vi "BinaryFile_input_output.vi"() -> ()   [LabVIEW 2018]
panel:
  out "웨이브폼 그래프":dbl[](graph)
  out "웨이브폼 차트":dbl(graph)
  in  "정지 버튼 2":bool
  in  "파일 경로(대화 상자 사용)":path
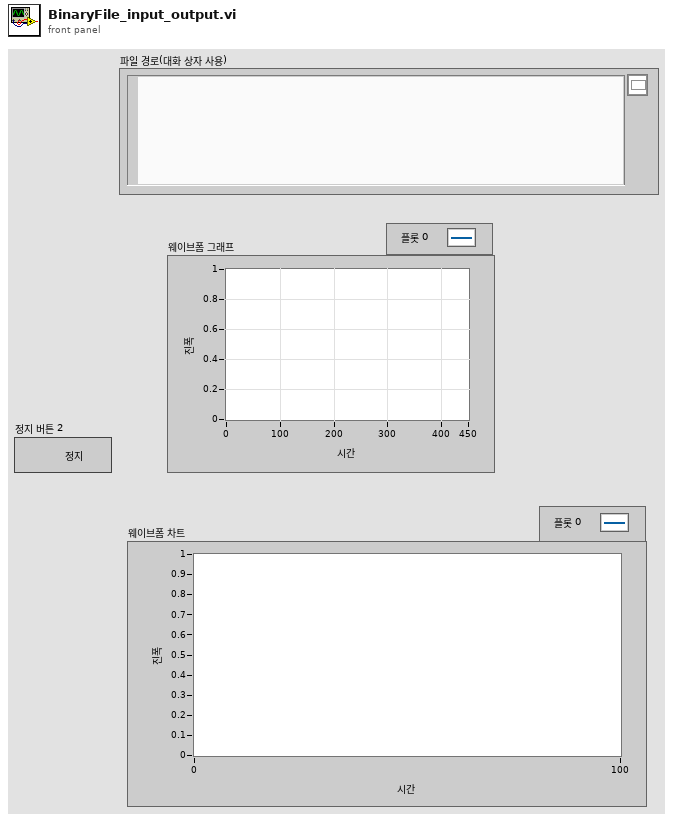
[diagram p1: front panel]
types:
  T1 = enum16{"open", "replace", "create", "open or create", "replace or create", "replace or create with confirmation"}
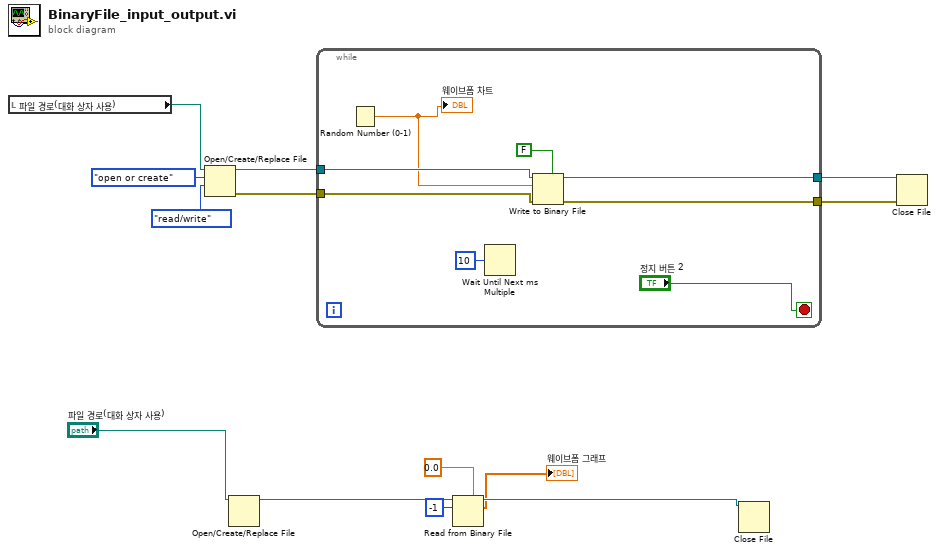
[diagram p0: block diagram]
diagram:
  n1 = local read "파일 경로(대화 상자 사용)"() -> (w11:path)
  n2 = Open/Create/Replace File(file path (use dialog)=w11, operation (0:open)=T1."open or create" ("동작(0:open)"), access (0:read/write)=enum16{"read/write", "read-only", "write-only"}."read/write" ("접근(0:읽기/쓰기)")) -> (refnum out=w13:refnum<file>, error out=w8:errorcluster)  [unwired: 3 in, 1 out]
  n3 = Open/Create/Replace File(file path (use dialog)="파일 경로(대화 상자 사용)") -> (refnum out=w5:refnum<file>)  [unwired: 5 in, 2 out]
  n4 = while {
    tunnel: w13 -> [w21]
    tunnel: [w20] -> w12
    tunnel: w8 -> [w17]
    tunnel: [w16] -> w7
    stop <- "정지 버튼 2" stop-if-true
    n5 = Random Number (0-1)() -> (number: 0 to 1=w18:dbl)
    "웨이브폼 차트" <- w18
    n6 = Wait Until Next ms Multiple(millisecond multiple=u32 10 ("ms 배수")) -> ()  [unwired: 1 out]
    n7 = Write to Binary File(file (use dialog)=w21, data=w18, error in=w17, 5:FALSE ("배열 또는 문자열 크기를 앞에 추가? (참)")) -> (refnum out=w20:refnum<file>, error out=w16:errorcluster)  [unwired: 2 in, 1 out]
  }
  n8 = Read from Binary File(5:0.0, 10:-1 ("카운트(1)"), 11:w5) -> (2:→"웨이브폼 그래프":dbl[], 3:w3:refnum<file>)  [unwired: 3 in, 2 out]
  n9 = Close File(refnum=w3) -> ()  [unwired: 1 in, 2 out]
  n10 = Close File(refnum=w12, error in=w7) -> ()  [unwired: 2 out]
